vi "BinaryTracer.vi"(0 "YActor in":refnum<class>, 1 "QueueData":T2, 2 "Target":string, 5 "Method Data output":refnum<class>, 7 "Reply Data":variant, 11 "Method Error in":errorcluster, 12 "Timing":T1, 13 "Method Call Error":errorcluster, 14 "Async Error":errorcluster) -> (15 "Method Error out":errorcluster)   [LabVIEW 2021, in "YActor.lvclass"]
uses:
  YActor.lvclass
  CmdCtrl.ctl
  AsyncErrorHandling.ctl
  CallMode.ctl
  tracing/RawTrace.ctl
  RawTrace.vi
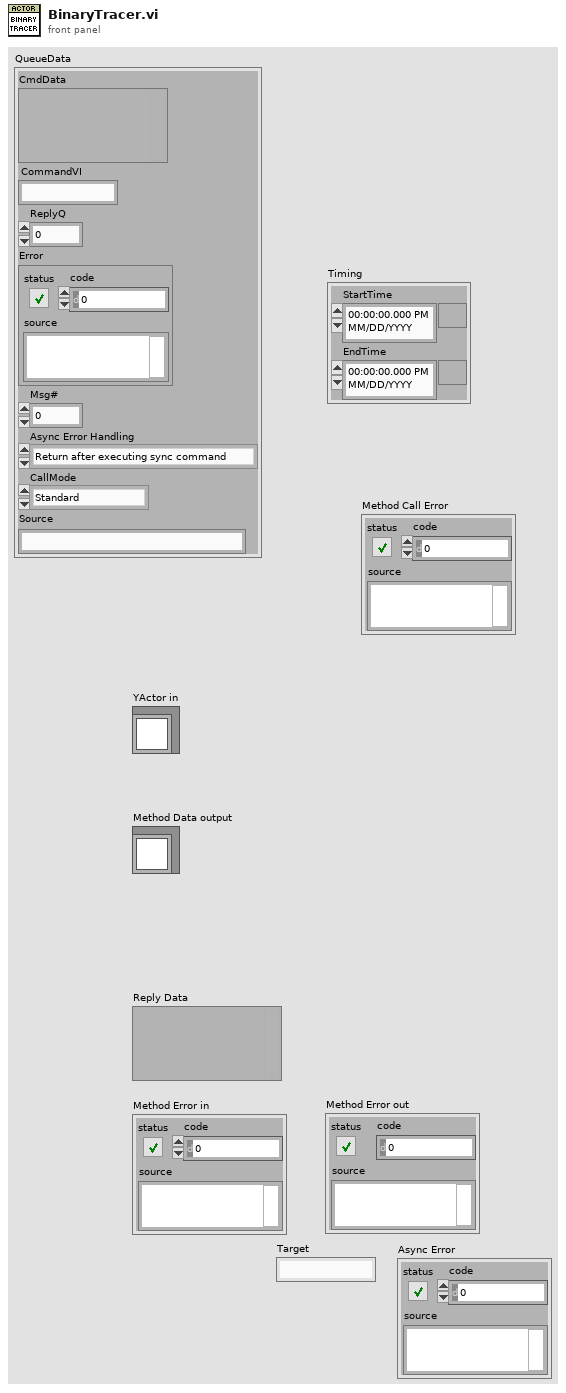
[diagram p1: front panel]
types:
  T1 = cluster{"StartTime":timestamp, "EndTime":timestamp}
  T2 = typedef "YActor.lvclass/CmdCtrl.ctl" = cluster{"CmdData":variant, "CommandVI":string, "ReplyQ":i64, "Error":errorcluster, "Msg#":u32, "Async Error Handling":T3, "CallMode":T4, "Source":string}
  T3 = typedef "YActor.lvclass/AsyncErrorHandling.ctl" = enum16{"Return after executing sync command", "Return before executing sync command", "Don't return error"}
  T4 = typedef "YActor.lvclass/CallMode.ctl" = enum16{"Standard", "Call&Collect"}
  T5 = typedef "YActor.lvclass/TraceDefinition.ctl" = enum16{"No Tracing", "Basic", "Basic + Method IO", "Basic + Method IO + Object in", "Basic + Method IO + Object IO"}
  T6 = typedef "YActor.lvclass/RawTrace.ctl" = cluster{"Time Stamp":timestamp, "QueueData":T2, "Target":string, "ActorInput":refnum<class>, "CmdData":variant, "ActorOutput":refnum<class>, "Reply Data":variant, "Execution Time":dbl, "VI server error":errorcluster, "Called VI error":errorcluster, "Async error":errorcluster}
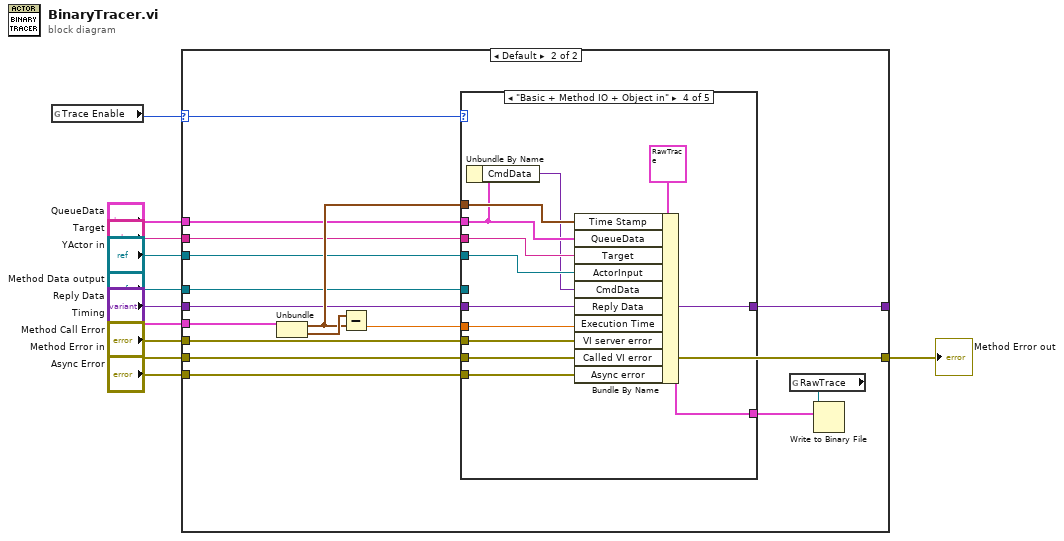
[diagram p0: block diagram]
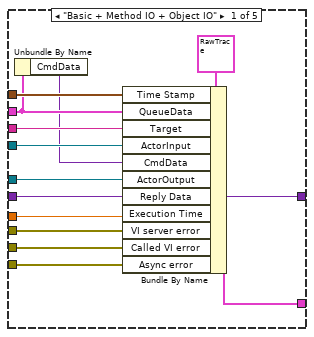
[diagram p3: hidden frame]
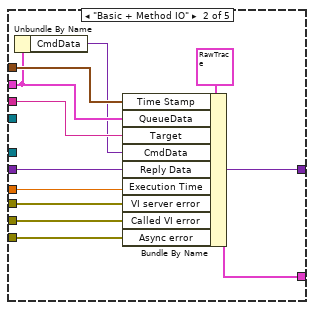
[diagram p4: hidden frame]
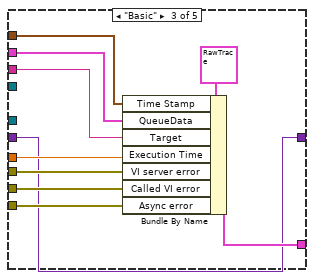
[diagram p5: hidden frame]
diagram:
  n1 = global read "RawTrace.vi" "Trace Enable"() -> (w2:T5)
  n2 = case shown="Default" w2 {
    selector: w2 -> [_ w16]
    tunnel: "Async Error" -> [_ w19]
    tunnel: "Method Error in" -> [w12 w14]
    tunnel: "QueueData" -> [_ w24]
    tunnel: "YActor in" -> [_ w22]
    tunnel: "Timing" -> [_ w20]
    tunnel: "Reply Data" -> [w13 w18]
    tunnel: "Target" -> [_ w23]
    tunnel: "Method Data output" -> [_ w21]
    tunnel: "Method Call Error" -> [_ w15]
    tunnel: [w13 w17] -> _
    tunnel: [w12 w14] -> w1
    frame "No Tracing" {
    }
    frame Default {
      n3 = Unbundle(w20) -> ("StartTime"=w25:timestamp, "EndTime"=w27:timestamp)
      n4 = Subtract(x=w27, y=w25) -> (x-y=w26:dbl)
      n5 = case shown="\"Basic + Method IO + Object in\"" w16 {
        tunnel: [w41 w52 w62 w74 _] -> w28
        tunnel: w26 -> [w40 w51 w61 w73 _]
        tunnel: w25 -> [w39 w50 w60 w66 _]
        tunnel: w24 -> [w31 w44 w59 w65 _]
        tunnel: w23 -> [w38 w49 w58 w72 _]
        tunnel: w22 -> [w34 _ _ w67 _]
        tunnel: w21 -> [w33 _ _ _ _]
        tunnel: w18 -> [w32 w45 w54 w68 w76]
        tunnel: w15 -> [w37 w48 w57 w71 _]
        tunnel: w14 -> [w36 w47 w56 w70 _]
        tunnel: w19 -> [w35 w46 w55 w69 _]
        tunnel: [w32 w45 w54 w68 w76] -> w17
        frame "Basic + Method IO + Object IO" {
          n6 = Unbundle By Name(w31) -> ("CmdData"=w30:variant)
          n7 = Bundle By Name(cluster=T6 {"Time Stamp"=timestamp(0 s since 1904-01-01), "QueueData"={"CmdData"=variant(string ""), "CommandVI"="", "ReplyQ"=0, "Error"={"status"=FALSE, "code"=0, "source"=""}, "Msg#"=0, "Async Error Handling"=enum."Return after executing sync command", "CallMode"=enum."Standard", "Source"=""}, "Target"="", "ActorInput"=refnum, "CmdData"=variant, "ActorOutput"=refnum, "Reply Data"=variant, "Execution Time"=0.0, "VI server error"={"status"=FALSE, "code"=0, "source"=""}, "Called VI error"={"status"=FALSE, "code"=0, "source"=""}, "Async error"={"status"=FALSE, "code"=0, "source"=""}} ("RawTrace"), "Time Stamp"=w39, "QueueData"=w31, "Target"=w38, "ActorInput"=w34, "CmdData"=w30, "ActorOutput"=w33, "Reply Data"=w32, "Execution Time"=w40, "VI server error"=w37, "Called VI error"=w36, "Async error"=w35) -> (w41:T6)
        }
        frame "Basic + Method IO" {
          n8 = Unbundle By Name(w44) -> ("CmdData"=w43:variant)
          n9 = Bundle By Name(cluster=T6 {"Time Stamp"=timestamp(0 s since 1904-01-01), "QueueData"={"CmdData"=variant(string ""), "CommandVI"="", "ReplyQ"=0, "Error"={"status"=FALSE, "code"=0, "source"=""}, "Msg#"=0, "Async Error Handling"=enum."Return after executing sync command", "CallMode"=enum."Standard", "Source"=""}, "Target"="", "ActorInput"=refnum, "CmdData"=variant, "ActorOutput"=refnum, "Reply Data"=variant, "Execution Time"=0.0, "VI server error"={"status"=FALSE, "code"=0, "source"=""}, "Called VI error"={"status"=FALSE, "code"=0, "source"=""}, "Async error"={"status"=FALSE, "code"=0, "source"=""}} ("RawTrace"), "Time Stamp"=w50, "QueueData"=w44, "Target"=w49, "CmdData"=w43, "Reply Data"=w45, "Execution Time"=w51, "VI server error"=w48, "Called VI error"=w47, "Async error"=w46) -> (w52:T6)
        }
        frame "Basic" {
          n10 = Bundle By Name(cluster=T6 {"Time Stamp"=timestamp(0 s since 1904-01-01), "QueueData"={"CmdData"=variant(string ""), "CommandVI"="", "ReplyQ"=0, "Error"={"status"=FALSE, "code"=0, "source"=""}, "Msg#"=0, "Async Error Handling"=enum."Return after executing sync command", "CallMode"=enum."Standard", "Source"=""}, "Target"="", "ActorInput"=refnum, "CmdData"=variant, "ActorOutput"=refnum, "Reply Data"=variant, "Execution Time"=0.0, "VI server error"={"status"=FALSE, "code"=0, "source"=""}, "Called VI error"={"status"=FALSE, "code"=0, "source"=""}, "Async error"={"status"=FALSE, "code"=0, "source"=""}} ("RawTrace"), "Time Stamp"=w60, "QueueData"=w59, "Target"=w58, "Execution Time"=w61, "VI server error"=w57, "Called VI error"=w56, "Async error"=w55) -> (w62:T6)
        }
        frame "Basic + Method IO + Object in" {
          n11 = Unbundle By Name(w65) -> ("CmdData"=w64:variant)
          n12 = Bundle By Name(cluster=T6 {"Time Stamp"=timestamp(0 s since 1904-01-01), "QueueData"={"CmdData"=variant(string ""), "CommandVI"="", "ReplyQ"=0, "Error"={"status"=FALSE, "code"=0, "source"=""}, "Msg#"=0, "Async Error Handling"=enum."Return after executing sync command", "CallMode"=enum."Standard", "Source"=""}, "Target"="", "ActorInput"=refnum, "CmdData"=variant, "ActorOutput"=refnum, "Reply Data"=variant, "Execution Time"=0.0, "VI server error"={"status"=FALSE, "code"=0, "source"=""}, "Called VI error"={"status"=FALSE, "code"=0, "source"=""}, "Async error"={"status"=FALSE, "code"=0, "source"=""}} ("RawTrace"), "Time Stamp"=w66, "QueueData"=w65, "Target"=w72, "ActorInput"=w67, "CmdData"=w64, "Reply Data"=w68, "Execution Time"=w73, "VI server error"=w71, "Called VI error"=w70, "Async error"=w69) -> (w74:T6)
        }
        frame "No Tracing" {
        }
      }
      n13 = global read "RawTrace.vi" "RawTrace"() -> (w29:refnum<file>)
      n14 = Write to Binary File(file (use dialog)=w29, data=w28) -> ()  [unwired: 4 in, 3 out]
    }
  }
  "Method Error out" <- w1
